vi "graphbuffer.vi"(8 "Reset":bool, 9 "history length":u16, 10 "Time":dbl format="%.2f", 11 "data":dbl[](array[numeric]) format="%.2f") -> (1 "data rate (Hz)":dbl format="%.2f", 2 "Mean":dbl[](array[numeric]) format="%.2f", 3 "Multiplot graph data":cluster{dbl[], dbl[]}[](array[cluster]) {"?" format="%.2f"; "?" format="%.2f"})   [LabVIEW 2019]
doc: "Takes an array containing one data point per channel and an arbitrary time. Creates data format required for an x-y plot with arbitrary data interval. Stores up to history number of data points per channel in a shift register.\nThis VI is reentrant meaning that it will hold different values if it is used at different places in a program. Thus more than one graph can be created!"
uses:
  <vilib>/Analysis/baseanly.llb/Mean (DBL).vi
  <vilib>/Analysis/NI_AALBase.lvlib
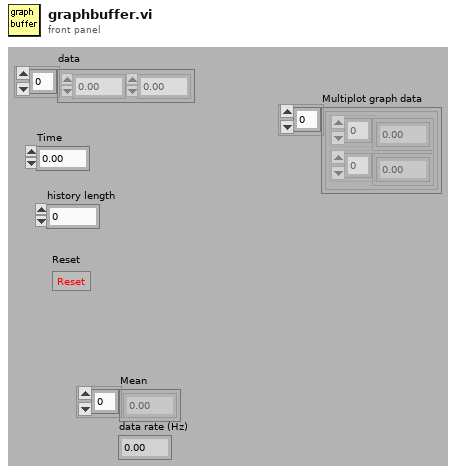
[diagram p1: front panel]
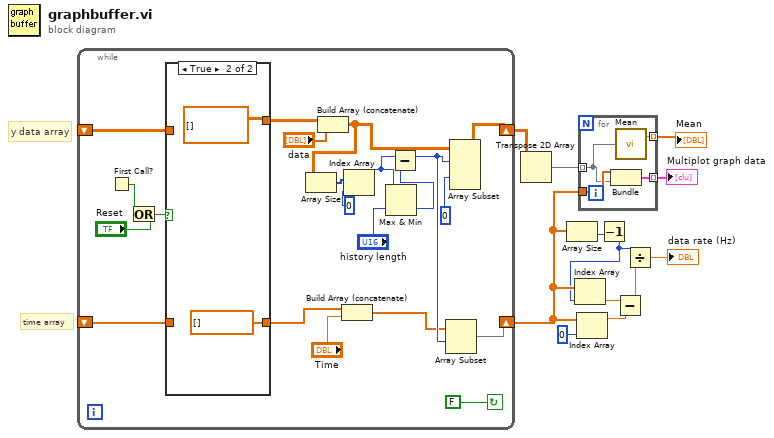
[diagram p0: block diagram]
diagram:
  # "time array"
  # "y data array"
  n1 = while {
    shift-left: _ -> [w22]
    shift-right: [w20] -> w8
    shift-left: _ -> [w32]
    shift-right: [w31] -> w12
    stop <- FALSE continue-if-true
    n2 = First Call?() -> (First Call?: T/F=w16:bool)
    n3 = Or(x=w16, y="Reset") -> (x .or. y?=w14:bool)
    n4 = case shown="True" w14 {
      tunnel: [w35 dbl[][] [] ("t")] -> w33
      tunnel: w32 -> [w35 _]
      tunnel: w22 -> [w34 _]
      tunnel: [w34 dbl[] []] -> w21
      frame False {
      }
      frame True {
      }
    }
    n5 = Build Array (concatenate)(w33, "data") -> (w28:dbl[][])
    n6 = Array Size(array=w28) -> (size(s)=w27:i32[])
    n7 = Build Array (concatenate)(w21, "Time") -> (w17:dbl[])
    n8 = Index Array(array=w27, index=0 ("Index")) -> (element=w23:i32)
    n9 = Max & Min(x=w23, y="history length") -> (min(x,y)=w19:i32)  [unwired: 1 out]
    n10 = Subtract(x=w23, y=w19) -> (x-y=w18:i32)
    n11 = Array Subset(array=w17, index=w18) -> (w20:dbl[])  [unwired: 1 in]
    n12 = Array Subset(array=w28, index (row)=w18, index (col)=0 ("Array Index")) -> (w31:dbl[][])  [unwired: 2 in]
  }
  n13 = Transpose 2D Array(2D array=w12) -> (transposed array=w10:dbl[][])
  n14 = Array Size(array=w8) -> (size(s)=w2:i32)
  n15 = Index Array(array=w8, index=0 ("Index")) -> (element=w5:dbl)
  n16 = for {
    tunnel: w10 -> [w39] mode=indexing
    tunnel: w8 -> [w41]
    tunnel: [w40] -> w11 mode=indexing
    tunnel: [w38] -> w9 mode=indexing
    n17 = Bundle(w41, w39) -> (w40:cluster{dbl[], dbl[]})  [unwired: 1 in]
    n18 = call-poly <vilib>:"Mean.vi"("X"=w39) -> ("mean"=w38:dbl)  [unwired: 1 out]
  }
  "Multiplot graph data" <- w11
  "Mean" <- w9
  n19 = Decrement(x=w2) -> (x-1=w1:i32)
  n20 = Index Array(array=w8, index=w1) -> (element=w6:dbl)
  n21 = Subtract(x=w6, y=w5) -> (x-y=w4:dbl)
  n22 = Divide(x=w1, y=w4) -> (x/y=→"data rate (Hz)":dbl)
